vi "ReadConfigArray.vi"(3 "error in (no error)":errorcluster, 4 "KeyArray":string[](array[string]), 5 "Section":string, 6 "Path":path) -> (0 "error out":errorcluster, 1 "Keys Found？":bool[](array[boolean]), 2 "ValueArray":string[](array[string]))   [LabVIEW 2013]
uses:
  <vilib>/Utility/config.llb/Read Key (String).vi
  <vilib>/Utility/config.llb/NI_LVConfig.lvlib
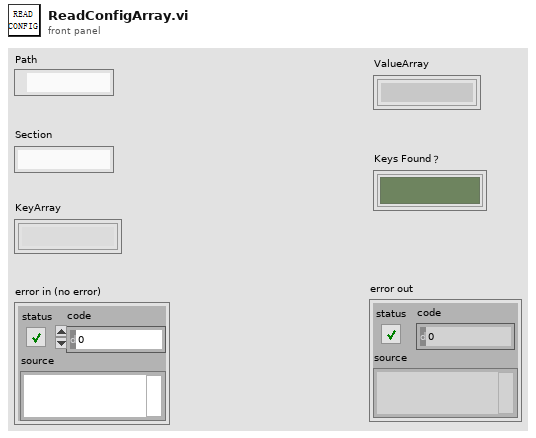
[diagram p1: front panel]
types:
  T1 = typedef "NI_LVConfig.lvlib/Config Data RefNum.ctl" = refnum<k1>
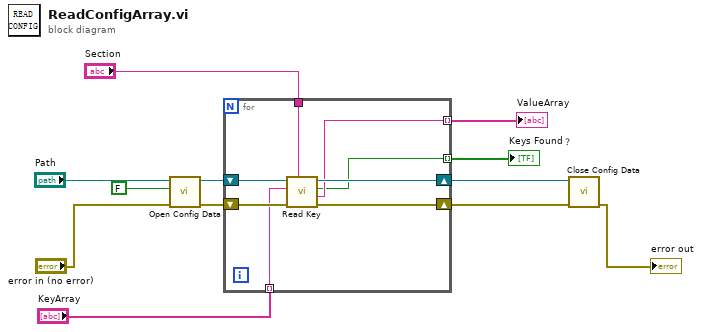
[diagram p0: block diagram]
diagram:
  n1 = call <vilib>:"Open Config Data.vi"("error in (no error)"="error in (no error)", "create file if necessary (T)"=FALSE, "configuration file path"="Path") -> ("error out"=w10:errorcluster, "refnum"=w8:T1)  [unwired: 6 in, 1 out]
  n2 = for {
    tunnel: "Section" -> [w16]
    shift-right: [w17] -> w7
    shift-left: w8 -> [w18]
    shift-right: [w19] -> w9
    shift-left: w10 -> [w20]
    tunnel: "KeyArray" -> [w15] mode=indexing
    tunnel: [w14] -> w2 mode=indexing
    tunnel: [w13] -> w1 mode=indexing
    n3 = call-poly <vilib>:"Read Key.vi"("section"=w16, "error in (no error)"=w20, "key"=w15, "refnum"=w18) -> ("error out"=w19:errorcluster, "value"=w14:string, "found?"=w13:bool, "refnum out"=w17:T1)  [unwired: 4 in]
  }
  "ValueArray" <- w2
  "Keys Found？" <- w1
  n4 = call <vilib>:"Close Config Data.vi"("error in (no error)"=w9, "refnum"=w7) -> ("error out"=→"error out":errorcluster)  [unwired: 8 in, 1 out]
